vi "FF-Restore Defaults.vi"() -> (8 "Parameters":T1)   [LabVIEW 2020]
uses:
  Typedefs/FF-Parameters.ctl
  Typedefs/FF-Stimulus.ctl
  Typedefs/FF-Response.ctl
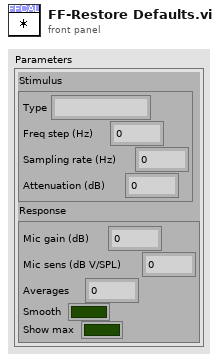
[diagram p1: front panel]
types:
  T1 = typedef "FF-Parameters.ctl" = cluster{"Stimulus":T2, "Response":T3}
  T2 = typedef "FF-Stimulus.ctl" = cluster{"Type":string, "Freq step (Hz)":dbl, "Sampling rate (Hz)":dbl, "Attenuation (dB)":dbl}
  T3 = typedef "FF-Response.ctl" = cluster{"Mic gain (dB)":dbl, "Mic sens (dB V/SPL)":dbl, "Averages":i32, "Smooth":bool, "Show max":bool}
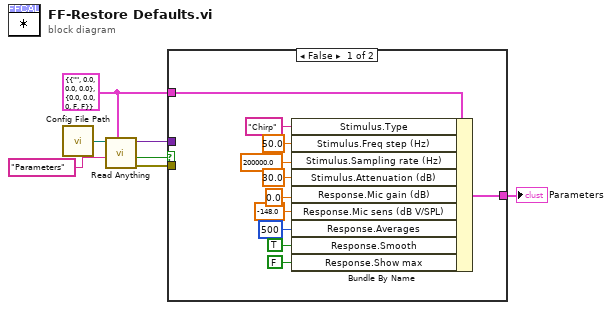
[diagram p0: block diagram]
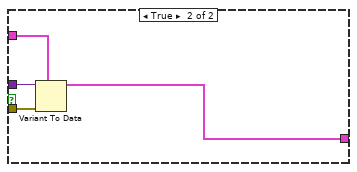
[diagram p2: hidden frame]
diagram:
  w2 = T1 {"Stimulus"={"Type"="", "Freq step (Hz)"=0.0, "Sampling rate (Hz)"=0.0, "Attenuation (dB)"=0.0}, "Response"={"Mic gain (dB)"=0.0, "Mic sens (dB V/SPL)"=0.0, "Averages"=0, "Smooth"=FALSE, "Show max"=FALSE}} ("Parameters")
  n1 = call "Config File Path.vi"() -> ("Default config file name"=w7:path)  [unwired: 1 in]
  n2 = call "Read Anything.vi"("Type of Anything"=w2, "Section Name (Name of \"Type of Anything\")"="Parameters" ("Section Name (Name of \"Type of Anything\")"), "Path (dialog)"=w7) -> ("Error Out"=w5:errorcluster, "Found?"=w4:bool, "Anything"=w3:variant)  [unwired: 6 in]
  n3 = case shown="False" w4 {
    tunnel: w5 -> [_ w22]
    tunnel: w3 -> [_ w21]
    tunnel: w2 -> [w18 w20]
    tunnel: [w17 w19] -> w1
    frame False {
      n4 = Bundle By Name(cluster=w18, "Stimulus.Type"="Chirp", "Stimulus.Freq step (Hz)"=50.0, "Stimulus.Sampling rate (Hz)"=200000.0, "Stimulus.Attenuation (dB)"=30.0, "Response.Mic gain (dB)"=0.0, "Response.Mic sens (dB V/SPL)"=-148.0, "Response.Averages"=500, "Response.Smooth"=TRUE, "Response.Show max"=FALSE) -> (w17:T1)
    }
    frame True {
      n5 = Variant To Data(error in=w22, type=w20, Variant=w21) -> (data=w19:T1)  [unwired: 1 out]
    }
  }
  "Parameters" <- w1
